vi "Read Message.vi"(8 "error in (no error)":errorcluster, 11 "RemoteControl.STM in":refnum<class "RemoteControl.STM.lvclass">) -> (0 "error out":errorcluster, 1 "Data":string, 2 "Command":string, 3 "RemoteControl.STM out":refnum<class "RemoteControl.STM.lvclass">, 4 "ID":string)   [LabVIEW 2019, in "RemoteControl.STM.lvclass"]
uses:
  RemoteControl.STM.lvclass
  C:/Program Files (x86)/National Instruments/LabVIEW 2019/user.lib/LevyLab/RemoteControl/RemoteControl/RemoteControl.lvclass
  <vilib>/NI/STM/TCP/TCP Read Options.ctl
  <userlib>/LevyLab/RemoteControl/RemoteControl/RemoteControl.lvclass/RemoteControl.ctl
  RemoteControl.STM.lvclass/RemoteControl.STM.ctl
  <vilib>/NI/STM/Connection Manager/TCP/TCP Connection Method.ctl
  <vilib>/NI/STM/TCP/Get Connection Reference (TCP).vi
  <vilib>/NI/STM/TCP/Read Message (TCP).vi
  <vilib>/Utility/error.llb/Error Cluster From Error Code.vi
  <vilib>/ErrorRing/Error Ring.xnode
  <vilib>/NI/STM/NI STM.lvlib
  <userlib>/LevyLab/RemoteControl/RemoteControl/RemoteControl.lvclass
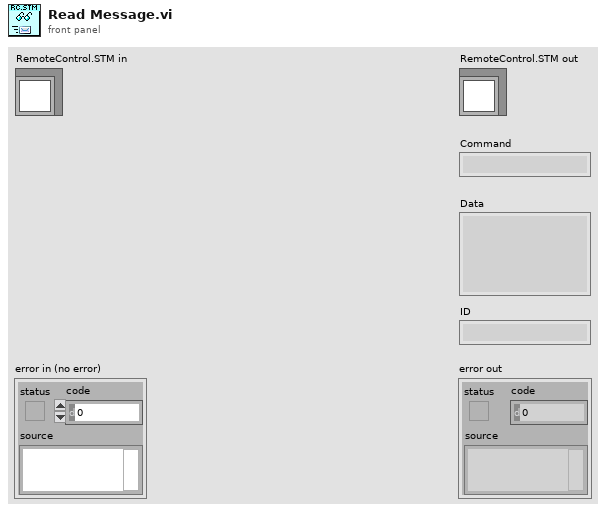
[diagram p1: front panel]
types:
  T1 = typedef "NI STM.lvlib/TCP Read Options.ctl" = cluster{"ignore timeout error":bool, "timeout ms (1000)":i32}
  T2 = typedef "NI STM.lvlib/TCP Connection Method.ctl" = enum16{"Initialize", "Add Connection", "Set Properties", "Get Connection(s)", "Remove Connection", "Remove All Connections", "Get Connection Count"}
  T3 = typedef "NI STM.lvlib/TCP Connection Info.ctl" = cluster{"connection ID":refnum<k5>, "meta data":T4[]}
  T4 = typedef "NI STM.lvlib/MetaDataElement.ctl" = string
  T5 = typedef "RemoteControl.lvlib/RemoteControl.lvclass/RC Process Type--Enum.ctl" = enum16{"Listener", "Server", "Client"}
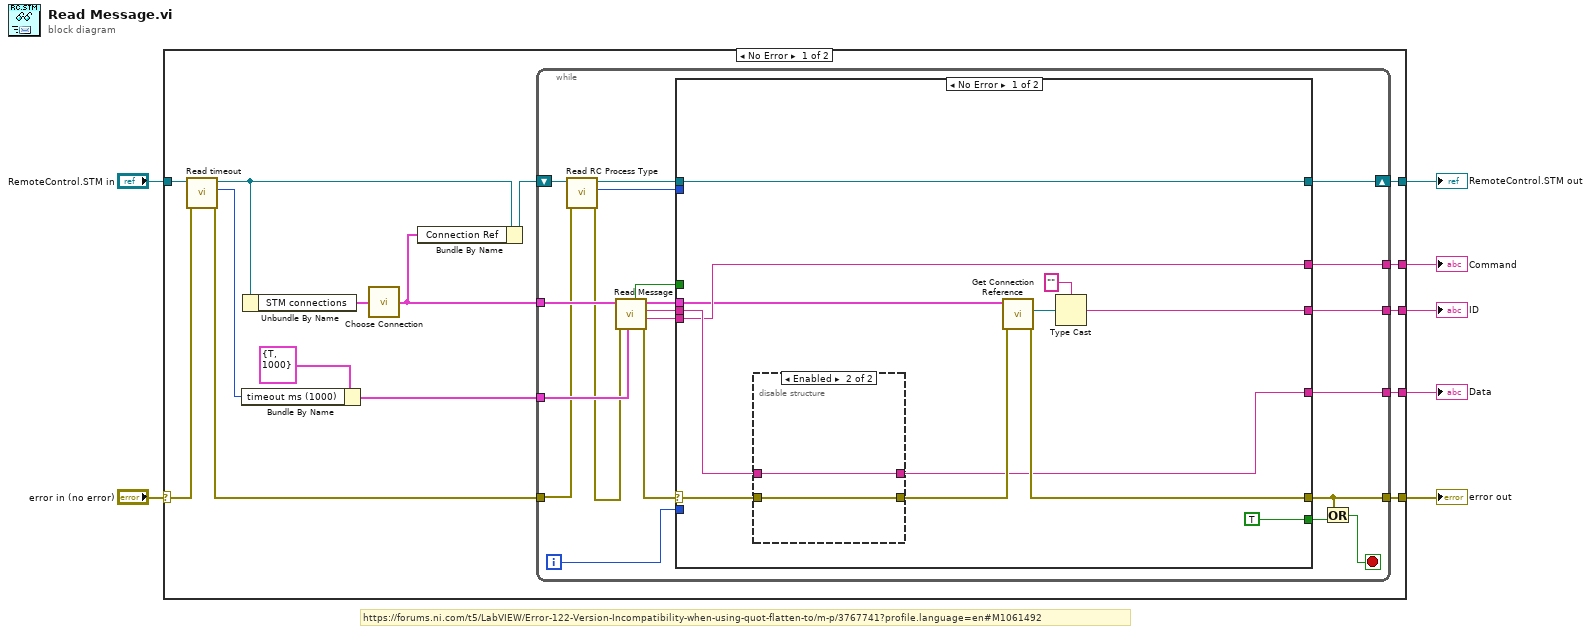
[diagram p0: block diagram]
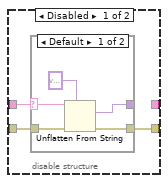
[diagram p2: hidden frame]
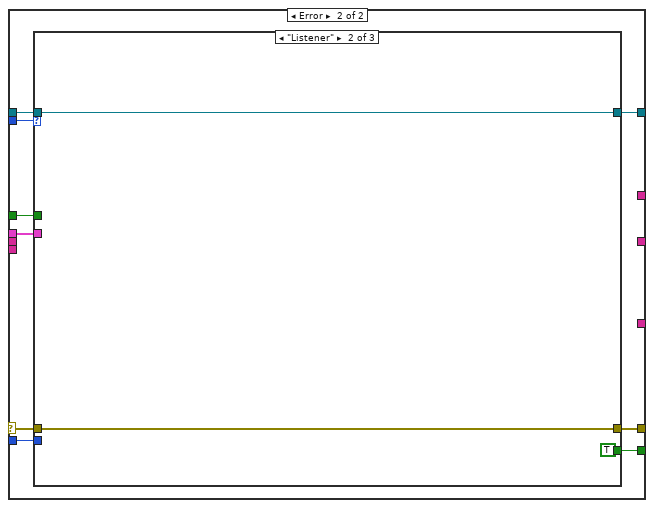
[diagram p4: hidden frame]
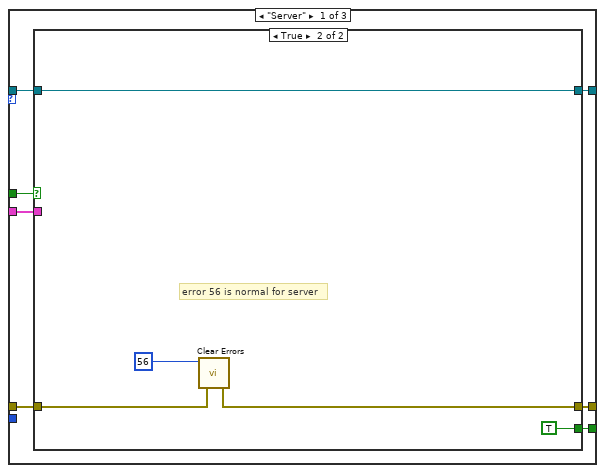
[diagram p5: hidden frame]
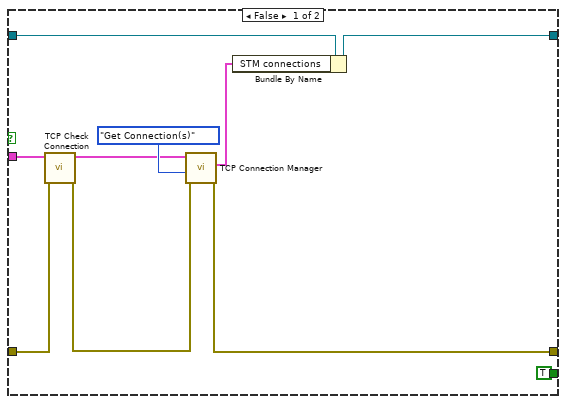
[diagram p6: hidden frame]
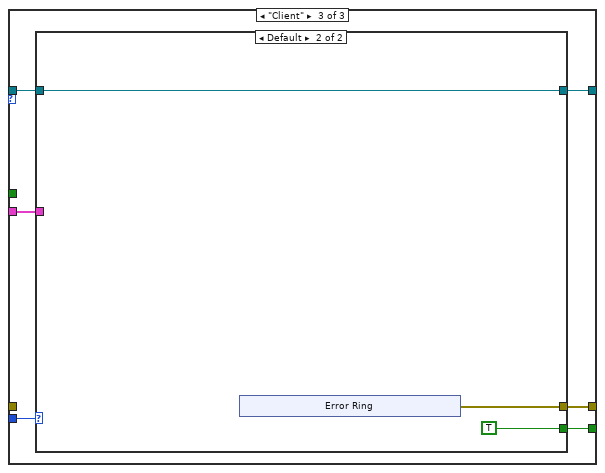
[diagram p7: hidden frame]
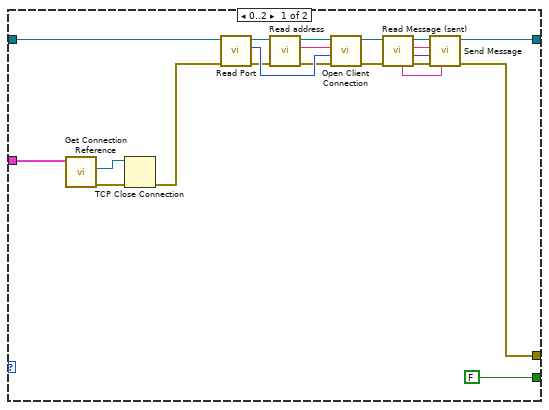
[diagram p8: hidden frame]
diagram:
  # "https://forums.ni.com/t5/LabVIEW/Error-122-Version-Incompatibility-when-using-quot-flatten-to/m-p/3767741?profile.language=en#M1061492"
  n1 = case shown="No Error" "error in (no error)" {
    selector: "error in (no error)" -> [w14 w134]
    tunnel: [w17 w134] -> w1
    tunnel: [w21 _] -> w5
    tunnel: [w18 _] -> w4
    tunnel: [w19 _] -> w2
    tunnel: [w16 w135] -> w3
    tunnel: "RemoteControl.STM in" -> [w15 w135]
    frame No Error {
      n2 = call <userlib>:"Read timeout.vi"("error in (no error)"=w14, "RemoteControl in"=w15) -> ("error out"=w12:errorcluster, "timeout"=w13:i32, "RemoteControl out"=w10:refnum<class "RemoteControl.STM.lvclass">)  [unwired: 7 in]
      n3 = Bundle By Name(cluster=T1 {"ignore timeout error"=TRUE, "timeout ms (1000)"=1000} ("options"), "timeout ms (1000)"=w13) -> (w20:T1)
      n4 = Unbundle By Name(w10) -> ("STM connections"=w11:T3[])
      n5 = call "Choose Connection.vi"("STM connections"=w11) -> ("Connection Ref"=w9:T3)
      n6 = Bundle By Name(cluster=w10, "Connection Ref"=w9) -> (w8:refnum<class "RemoteControl.STM.lvclass">)
      n7 = while {
        tunnel: w9 -> [w42]
        tunnel: [w36] -> w21
        tunnel: w20 -> [w39]
        tunnel: [w38] -> w19
        tunnel: [w37] -> w18
        shift-right: [w33] -> w16
        shift-left: w8 -> [w31]
        tunnel: w12 -> [w29]
        tunnel: [w23] -> w17
        i -> [w34]
        stop <- w24 stop-if-true
        n8 = call <userlib>:"Read RC Process Type.vi"("error in (no error)"=w29, "RemoteControl in"=w31) -> ("error out"=w28:errorcluster, "RC Process Type"=w32:T5, "RemoteControl out"=w30:refnum<class "RemoteControl.STM.lvclass">)  [unwired: 7 in]
        n9 = call-poly <vilib>:"Read Message.vi"("options"=w39, "error in"=w28, "connection info in"=w42) -> ("error out"=w27:errorcluster, "name"=w35:T4, "data string"=w41:string, "connection info out"=w40:T3, "timed out?"=w26:bool)  [unwired: 3 in, 1 out]
        n10 = case shown="No Error" w27 {
          selector: w27 -> [w45 w67]
          tunnel: w41 -> [w47 _]
          tunnel: w40 -> [w44 w66]
          tunnel: [w51 _] -> w38
          tunnel: [w43 _] -> w37
          tunnel: [w50 w74] -> w23
          tunnel: [w46 _] -> w36
          tunnel: w35 -> [w46 _]
          tunnel: w34 -> [_ w73]
          tunnel: [TRUE w69] -> w25
          tunnel: [w48 w71] -> w33
          tunnel: w30 -> [w48 w72]
          tunnel: w32 -> [_ w68]
          tunnel: w26 -> [_ w70]
          frame No Error {
            n11 = disable-structure shown="Enabled" {
              disable-tunnel: [w57 w64] -> w52
              disable-tunnel: w47 -> [w56 w65]
              disable-tunnel: w45 -> [w55 w64]
              disable-tunnel: [_ w65] -> w43
              frame Disabled {
                n12 = case shown="Default" w56 {
                  selector: w56 -> [w62 _]
                  tunnel: w55 -> [w60 w63]
                  tunnel: [w59 w63] -> w57
                  tunnel: [w58 _] -> _
                  frame Default {
                    n13 = Unflatten From String(type=variant, binary string=w62, error in (no error)=w60) -> (value=w58:variant, error out=w59:errorcluster)  [unwired: 2 in, 1 out]
                  }
                  frame "" {
                  }
                }
              }
              frame Enabled {
              }
            }
            n14 = call-poly <vilib>:"Get Connection Reference.vi"("error in"=w52, "connection info in"=w44) -> ("error out"=w50:errorcluster, "connection ID out"=w54:refnum<k5>)  [unwired: 7 in, 1 out]
            n15 = Type Cast(type="", x=w54) -> (*(type *) &x=w51:string)
          }
          frame Error {
            n16 = case shown="\"Listener\"" w68 {
              tunnel: [w79 w98 w103] -> w74
              tunnel: w73 -> [_ _ w104]
              tunnel: w72 -> [w76 w99 w105]
              tunnel: [w75 w99 w100] -> w71
              tunnel: w67 -> [w80 w98 _]
              tunnel: w66 -> [w77 _ w101]
              tunnel: w70 -> [w81 _ _]
              tunnel: [w78 TRUE w102] -> w69
              frame "Server" {
                n17 = case shown="True" w81 {
                  tunnel: w80 -> [w90 w95]
                  tunnel: [w83 w94] -> w79
                  tunnel: [TRUE TRUE] -> w78
                  tunnel: w77 -> [w91 _]
                  tunnel: w76 -> [w85 w92]
                  tunnel: [w84 w92] -> w75
                  frame False {
                    n18 = call <vilib>:"TCP Check Connection.vi"("error in"=w90, "connection in"=w91) -> ("error out"=w86:errorcluster, "connection out"=w87:T3)  [unwired: 7 in, 1 out]
                    n19 = call <vilib>:"TCP Connection Manager.vi"("error in"=w86, "method"=TCP_Connection_Method."Get Connection(s)", "connection in"=w87) -> ("error out"=w83:errorcluster, "all connections"=w89:T3[])  [unwired: 3 in, 4 out]
                    n20 = Bundle By Name(cluster=w85, "STM connections"=w89) -> (w84:refnum<class "RemoteControl.STM.lvclass">)
                  }
                  frame True {
                    # "error 56 is normal for server"
                    n21 = call <vilib>:"Clear Errors.vi"("error in (no error)"=w95, "specific error code to clear (0: all)"=56) -> ("error out"=w94:errorcluster)  [unwired: 4 in, 1 out]
                  }
                }
              }
              frame "Listener" {
              }
              frame "Client" {
                n22 = case shown="Default" w104 {
                  tunnel: [w125 w128] -> w103
                  tunnel: w105 -> [w108 w129]
                  tunnel: [w126 w129] -> w100
                  tunnel: [FALSE TRUE] -> w102
                  tunnel: w101 -> [w109 _]
                  frame 0..2 {
                    n23 = call-poly <vilib>:"Get Connection Reference.vi"("connection info in"=w109) -> ("error out"=w110:errorcluster, "connection ID out"=w111:refnum<k5>)  [unwired: 8 in, 1 out]
                    n24 = TCP Close Connection(connection ID=w111, error in (no error)=w110) -> (error out=w107:errorcluster)  [unwired: 1 in, 1 out]
                    n25 = call-dynamic "Read Port.vi"("error in (no error)"=w107, "RemoteControl in"=w108) -> ("error out"=w114:errorcluster, "Port"=w115:u16, "RemoteControl out"=w118:refnum<class "RemoteControl.STM.lvclass">)  [unwired: 7 in]
                    n26 = call-dynamic "Read address.vi"("error in (no error)"=w114, "RemoteControl in"=w118) -> ("error out"=w113:errorcluster, "address"=w116:string, "RemoteControl out"=w117:refnum<class "RemoteControl.STM.lvclass">)  [unwired: 7 in]
                    n27 = call-dynamic "Open Client Connection.vi"("error in (no error)"=w113, "Port"=w115, "address"=w116, "RemoteControl.STM in"=w117) -> ("error out"=w119:errorcluster, "RemoteControl.STM out"=w120:refnum<class "RemoteControl.STM.lvclass">)  [unwired: 6 in]
                    n28 = call <userlib>:"Read Message (sent).vi"("error in (no error)"=w119, "RemoteControl in"=w120) -> ("error out"=w122:errorcluster, "Data (Sent)"=w106:variant, "Command (Sent)"=w123:string, "RemoteControl out"=w124:refnum<class "RemoteControl.STM.lvclass">, "ID (Sent)"=w121:string)  [unwired: 5 in]
                    n29 = call-dynamic "Send Message.vi"("ID"=w121, "error in (no error)"=w122, "Data"=w106, "Command"=w123, "RemoteControl.STM in"=w124) -> ("error out"=w125:errorcluster, "RemoteControl.STM out"=w126:refnum<class "RemoteControl.STM.lvclass">)  [unwired: 5 in]
                  }
                  frame Default {
                    n30 = xnode "Error Ring"() -> ("error out"=w128:errorcluster)
                  }
                }
              }
            }
          }
        }
        n31 = Or(x=w23, y=w25) -> (x .or. y?=w24:bool)
      }
    }
    frame Error {
    }
  }
  "error out" <- w1
  "RemoteControl.STM out" <- w3
  "ID" <- w2
  "Data" <- w4
  "Command" <- w5
